vi "GestureOLED.vi"() -> ()   [LabVIEW 2024]
uses:
  Driver/Public/Digital Pull Direction.ctl
  4ccb7be8-d2ac-470e-b164-43973984285f.vi
  4331f14a-4e11-4a16-bb0d-2e9d18c5c6a1.vi
  51c12f6e-4a21-4d98-9fb3-1a2e6b8270e3.vi
  d8ff4ad1-6435-4902-b67c-6ac0edf8525d.vi
  64x128OLED/Public/InitialiseOLED.vi
  64x128OLED/Public/GetPicture.vi
  64x128OLED/Public/BuildMessagesFromPicture.vi
  Driver/CTIPicoVISA.lvlib
  64x128OLED/OLEDI2CMessageGenerator.lvlib
panel:
  out "Stopped":bool
  out "Numeric":i32
  out "2D Picture":picture
  out "loop":i32
  out "Identity":T1
  out "Init Data":string
  in  "stop":bool
  in  "VISA resource name in":refnum<visa-resource-name>="COM7"
  out "error out":errorcluster
  # "https://www.seeedstudio.com/Grove-Gesture-PAJ7620U2.html"
  # "https://wiki.seeedstudio.com/Grove-OLED-Display-0.96-SSD1315/"
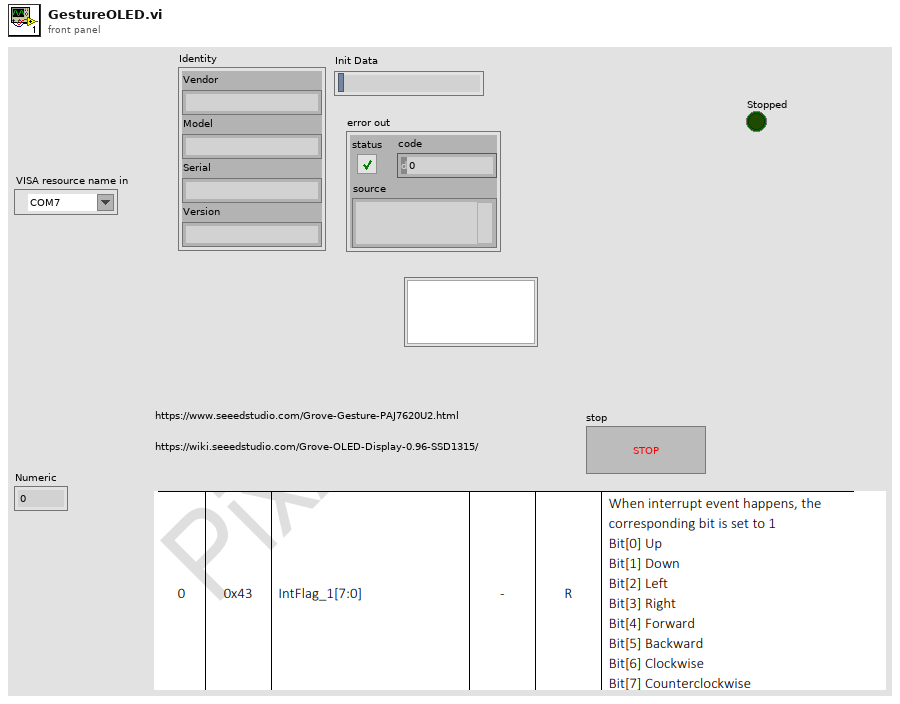
[diagram p1: front panel]
types:
  T1 = cluster{"Vendor":string, "Model":string, "Serial":string, "Version":string}
  T2 = cluster{"image type":i32, "image depth":i32, "image":u8[], "mask":u8[], "colors":u32[], "Rectangle":cluster{"left":i16, "top":i16, "right":i16, "bottom":i16}}
  T3 = typedef "CTIPicoVISA.lvlib/Digital Pull Direction.ctl" = enum16{"None", "Up", "Down", "Both"}
  T4 = cluster{"image type":i32, "image depth":i32, "image":u8[], "mask":u8[], "colors":u32[], "Rectangle":cluster{"left":i16, "top":i16, "right":i16, "bottom":i16}}[]
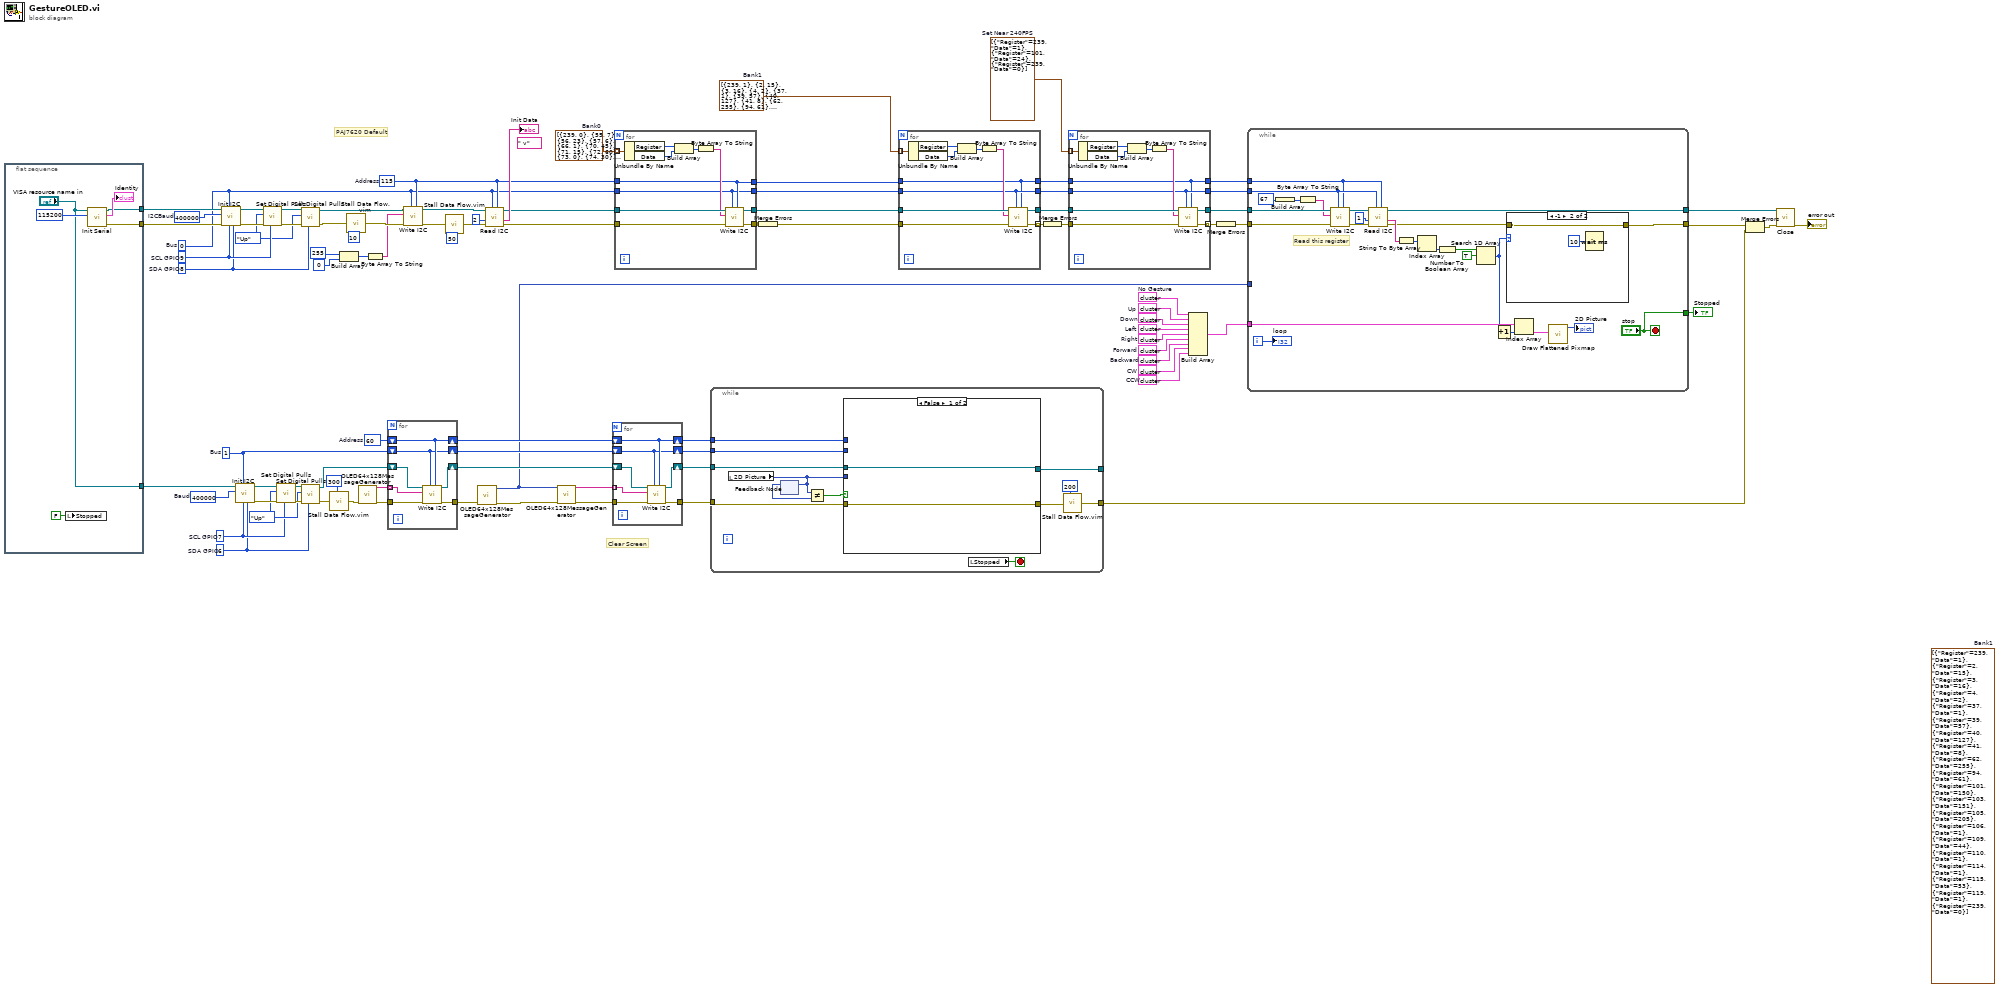
[diagram p0: block diagram]
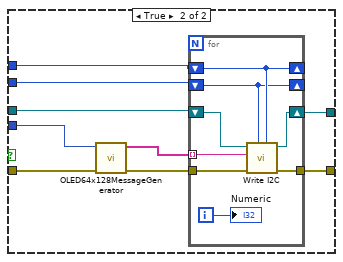
[diagram p2: hidden frame]
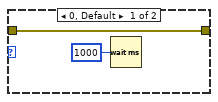
[diagram p3: hidden frame]
diagram:
  w1 = T2 {"image type"=0, "image depth"=8, "image"=array[8192 elements], "mask"=[], "colors"=[16777215, 15461356, 16579836, 11513775, 8158332, 13421772, 13816530, 0, 921102, 15329769, 8553090, 3421236, 15461355, 14935011, 1447446, 10000536, 1052688, 14803425, 15921906, 15000804, 13684944, 15856113, 16645629, 15658734, 3552822, 4079166, 11119017, 8289918, 4276545, 1052687, 395014, 7829367, 12171705, 15527148, 11645361, 65793, 131586, 2763306, 10987431, 16119285, 16316664, 6316128, 197379, 6447714, 14277081, 13158600, 6645093, 11316396, 13224393, 11184810, 6250335, 263172, 2171169, 13948116, 8092539, 10066329, 16250871, 12829635, 6118749, 2434341, 14013909, 16711422, 13750737, 8816262, 9868950, 14869218, 9474192, 4144959, 10658466, 3750201, 4934475, 15987699, 10724259, 328965, 9934743, 15790320, 12237498, 5592405, 15263976, 16185078, 6842472, 789516, 13487565, 7763574, 3815994, 16382457, 16514043, 5921370, 789515, 13092807, 12566463, 3684408, 12632256, 3355443, 11053224, 15592941, 14737632, 14145495, 5197647, 7697781, 14540253, 9408399, 16448250, 12698049, 12369084, 11579568, 14474460, 1644825, 5131854, 15066597, 3158320, 14671839, 4539717, 13355979, 13027014, 11382189, 10197915, 7105644, 15724527, 6974058, 7960953, 9276813, 8026746, 9342606, 4210752, 12303291, 11250603, 13882323, 11776947, 9013641, 8355711, 8882055, 11711154, 15527405, 14343133, 13553358, 14342874, 1907997, 7434609, 394758, 2368548, 5460819, 6710886, 4605510, 6776679, 12895428, 657930, 2302755, 5066061, 4473924, 3158064, 8618883, 2236962, 9079434, 4408131, 14079702, 13290186, 9211020, 7039851, 13619151, 5789784, 4342338, 5987163, 460551, 6513507, 855309, 5000268, 1315860, 12040119, 5526612, 9539985, 4802889, 12105912, 3092271, 986895, 8224125, 9605778, 2829099, 1776411, 7566195, 1381653, 2500134, 15395562, 0, 0, 0, 0, 0, 0, 0, 0, 0, 0, 0, 0, 0, 0, 0, 0, 0, 0, 0, 0, 0, 0, 0, 0, 0, 0, 0, 0, 0, 0, 0, 0, 0, 0, 0, 0, 0, 0, 0, 0, 0, 0, 0, 0, 0, 0, 0, 0, 0, 0, 0, 0, 0, 0, 0, 0, 0, 0, 0, 0, 0, 0, 0, 0, 0, 0, 0, 0, 0, 0, 0, 0, 0], "Rectangle"={"left"=0, "top"=0, "right"=128, "bottom"=64}}  # CCW
  w2 = T2 {"image type"=0, "image depth"=8, "image"=array[8192 elements], "mask"=[], "colors"=[16777215, 15461356, 13421772, 8158332, 11513775, 16579836, 15329769, 921102, 0, 13816530, 15461355, 3421236, 8553090, 10000536, 1447446, 14935011, 16645629, 15856113, 13684944, 15000804, 15921906, 14803425, 1052688, 15527148, 12171705, 7829367, 4079166, 395014, 1052687, 4276545, 8289918, 11119017, 3552822, 15658734, 16119285, 10987431, 2763306, 131586, 65793, 11645361, 14277081, 6447714, 197379, 6316128, 16316664, 13948116, 2171169, 263172, 6250335, 11184810, 13224393, 13158600, 11316396, 6645093, 14013909, 2434341, 6118749, 12829635, 16250871, 10066329, 8092539, 4144959, 9474192, 14869218, 9868950, 8816262, 13750737, 16711422, 9934743, 328965, 10724259, 15987699, 4934475, 3750201, 10658466, 789516, 6842472, 16185078, 15263976, 5592405, 12237498, 15790320, 16382457, 3815994, 7763574, 13487565, 5921370, 16514043, 13092807, 789515, 12566463, 12632256, 3684408, 3355443, 15592941, 11053224, 7697781, 5197647, 14145495, 14737632, 12698049, 16448250, 9408399, 14540253, 5131854, 1644825, 14474460, 11579568, 12369084, 13355979, 4539717, 14671839, 3158320, 15066597, 10197915, 11382189, 13027014, 6974058, 15724527, 7105644, 9342606, 8026746, 9276813, 7960953, 12303291, 4210752, 11250603, 11711154, 8882055, 8355711, 9013641, 11776947, 13882323, 15527405, 14343133, 1907997, 8750469, 14342874, 6776679, 12895428, 7368816, 3092271, 8947848, 3618615, 5066061, 12040119, 4802889, 5789784, 5723991, 526344, 14079702, 13290186, 3487029, 13619151, 9803157, 14408667, 394758, 460551, 4408131, 2894892, 5000268, 986895, 5658198, 12105912, 6513507, 7566195, 1973790, 5526612, 2829099, 1776411, 15395562, 0, 0, 0, 0, 0, 0, 0, 0, 0, 0, 0, 0, 0, 0, 0, 0, 0, 0, 0, 0, 0, 0, 0, 0, 0, 0, 0, 0, 0, 0, 0, 0, 0, 0, 0, 0, 0, 0, 0, 0, 0, 0, 0, 0, 0, 0, 0, 0, 0, 0, 0, 0, 0, 0, 0, 0, 0, 0, 0, 0, 0, 0, 0, 0, 0, 0, 0, 0, 0, 0, 0, 0, 0, 0, 0, 0, 0, 0, 0, 0, 0, 0, 0, 0, 0], "Rectangle"={"left"=0, "top"=0, "right"=128, "bottom"=64}}  # CW
  w3 = T2 {"image type"=0, "image depth"=8, "image"=array[8192 elements], "mask"=[], "colors"=[16777215, 16250871, 15724527, 14935011, 14079702, 13421772, 12961221, 15000804, 15921906, 14145495, 11842740, 9342606, 6381921, 3026478, 0, 2960685, 6447714, 9408399, 15395562, 8092539, 3421236, 3487029, 8026746, 11645361, 5066061, 256, 11579568, 16514043, 6513507, 13487565, 16514299, 15856113, 10658466, 1118481, 263172, 263428, 1052944, 10724259, 8684676, 131586, 15198183, 7434609, 65793, 7368816, 723979, 6513763, 2631976, 10066585, 12237754, 12171961, 12171960, 4539973, 14935267, 4605766, 9013640, 15790320, 9013641, 9211275, 15987699, 15987955, 9277068, 11776947, 9803156, 16119285, 16316664, 262916, 10527135, 16382457, 10790308, 11053480, 11776946, 16645885, 16711422, 11908789, 12040375, 2434597, 10198170, 12895683, 12895684, 13224649, 16711678, 13224393, 12961476, 10395550, 2566184, 4934731, 15066596, 13619407, 13422028, 16382456, 16316920, 13487564, 13684943, 15066597, 9013897, 13882579, 13553613, 13488077, 13816529, 9671571, 16185078, 9868950, 10724258, 16448250, 11316396, 16579835, 197379, 11908532, 11777203, 12369083, 12566463, 12763841, 132098, 7960953, 2698025, 13092806, 13092807, 3026733, 328965, 3224112, 10395806, 10527136, 3421492, 328709, 6513251, 986895, 16579836, 8618883, 7303023, 15329769, 15132390, 657930, 1118737, 3026477, 14211288, 13355979, 14013909, 16645629, 5658198, 1513239, 8224125, 5526612, 2434341, 7039851, 13027014, 4868682, 394758, 11447982, 9276813, 10066329, 16053492, 9539985, 7500402, 10526880, 4079166, 6974058, 11908533, 12303291, 6908265, 2894892, 3684408, 14869218, 2171169, 4737096, 3552822, 3355443, 3881787, 3815994, 15658734, 14606046, 5723991, 3750201, 2565927, 10329501, 10263708, 10855845, 7895160, 8882055, 13816530, 8487297, 13684944, 2829099, 1842204, 4013373, 6579300, 1447446, 8750469, 5131854, 2368548, 3618615, 10461087, 9474192, 14277081, 11184810, 1315860, 6184542, 8947848, 789516, 7763574, 1381653, 12763842, 12105912, 5987163, 1579032, 6776679, 15527148, 1907997, 0, 0, 0, 0, 0, 0, 0, 0, 0, 0, 0, 0, 0, 0, 0, 0, 0, 0, 0, 0, 0, 0, 0, 0, 0, 0, 0, 0, 0, 0, 0, 0, 0, 0, 0, 0, 0, 0, 0, 0, 0, 0, 0, 0, 0, 0, 0, 0, 0], "Rectangle"={"left"=0, "top"=0, "right"=128, "bottom"=64}}  # Backward
  w4 = T2 {"image type"=0, "image depth"=8, "image"=array[8192 elements], "mask"=[], "colors"=[16777215, 16250871, 15724527, 15000804, 14079702, 13421772, 12961221, 13355979, 14013909, 14935011, 15921906, 14145495, 11842740, 9408399, 6447714, 3026477, 0, 3026478, 9342606, 14211288, 15395562, 8026746, 3487029, 3421236, 11645361, 5066061, 16514043, 13487565, 6513507, 15856113, 10724259, 657930, 263172, 1118737, 10658466, 8684676, 131586, 8618883, 15329769, 15198183, 7368816, 65793, 7303023, 15132390, 16579836, 256, 1118481, 986895, 6513251, 11579568, 197379, 328965, 3224112, 10395806, 10527136, 3421492, 328709, 2698025, 13092806, 13092807, 3026733, 12566463, 12763841, 132098, 7960953, 12369083, 16711422, 11908532, 11777203, 11776947, 11316396, 16579835, 10724258, 16448250, 6381921, 2960685, 10066585, 9868950, 9671571, 16185078, 9013897, 13882579, 13553613, 13488077, 13816529, 9013641, 4934731, 15066596, 13619407, 13422028, 16382456, 16316920, 13487564, 13684943, 15066597, 2434597, 10198170, 12895683, 12895684, 11908789, 13224649, 16711678, 13224393, 12961476, 10395550, 2566184, 12040375, 11776946, 16645885, 11053480, 16514299, 10527135, 16382457, 10790308, 9803156, 16119285, 16316664, 262916, 9211275, 15987699, 15987955, 9277068, 9013640, 15790320, 4539973, 14935267, 4605766, 2631976, 12237754, 12171961, 12171960, 6513763, 723979, 7434609, 263428, 1052944, 8092539, 16645629, 15263976, 1776411, 5658198, 6052956, 3355443, 2434341, 15527148, 5395026, 10197915, 7105644, 9474192, 15461355, 8750469, 8553090, 8289918, 8882055, 11908533, 7895160, 3618615, 12698049, 7039851, 4013373, 11053224, 723723, 5329233, 1315860, 1513239, 14671839, 12829635, 3289650, 5460819, 14606046, 11513775, 2763306, 7566195, 6776679, 5921370, 3552822, 5855577, 5789784, 921102, 7171437, 7237230, 11184810, 2368548, 7763574, 13027014, 4276545, 15658734, 1579032, 14803425, 1907997, 2565927, 6579300, 10855845, 11711154, 6908265, 3750201, 8224125, 8816262, 2500134, 10921638, 460551, 6316128, 6118749, 5723991, 14277081, 12632256, 7829367, 2631720, 1644825, 10329501, 4934475, 14474460, 3947580, 4539717, 10132122, 1710618, 5592405, 14737632, 5131854, 10790052, 526344, 4605510, 3815994, 12303291, 2894892, 3881787, 4079166, 5197647, 6184542, 10987431, 12040119, 9737364, 855309, 10000536, 4737096, 13750737, 789516, 5000268, 8355711, 0, 0, 0, 0, 0, 0, 0, 0, 0, 0, 0, 0, 0, 0, 0, 0, 0], "Rectangle"={"left"=0, "top"=0, "right"=128, "bottom"=64}}  # Forward
  w6 = T2 {"image type"=0, "image depth"=24, "image"=array[24576 elements], "mask"=[], "colors"=[], "Rectangle"={"left"=0, "top"=0, "right"=128, "bottom"=64}}  # Right
  w7 = T2 {"image type"=0, "image depth"=24, "image"=array[24576 elements], "mask"=[], "colors"=[], "Rectangle"={"left"=0, "top"=0, "right"=128, "bottom"=64}}  # Left
  w8 = T2 {"image type"=0, "image depth"=24, "image"=array[24576 elements], "mask"=[], "colors"=[], "Rectangle"={"left"=0, "top"=0, "right"=128, "bottom"=64}}  # Down
  w9 = T2 {"image type"=0, "image depth"=24, "image"=array[24576 elements], "mask"=[], "colors"=[], "Rectangle"={"left"=0, "top"=0, "right"=128, "bottom"=64}}  # Up
  w10 = T2 {"image type"=0, "image depth"=8, "image"=array[8192 elements], "mask"=[], "colors"=[16777215, 16645629, 14869218, 7237230, 16579836, 14342874, 15592941, 11316396, 3750201, 10395294, 1776411, 5921370, 11250603, 16514043, 7500402, 6513507, 11447982, 13619151, 11776947, 0, 13158600, 5592405, 13224393, 15790320, 12171705, 16711422, 5658198, 14474460, 15658734, 5789784, 2368548, 13948116, 14277081, 13882323, 8750469, 8421504, 16316664, 12237498, 12369084, 14935011, 12105912, 11711154, 12763842, 15066597, 12303291, 11579568, 13421772, 9737364, 9803157, 15198183, 4671303, 13750737, 12434877, 16382457, 5329233, 4737096, 5460819, 5723991, 15856113, 16448250, 11053224, 14540253, 12698049, 13027014, 6250335, 13487565, 131586, 7105644, 65793, 1907997, 13355979, 15921906, 8816262, 11184810, 460551, 4473924, 5131854, 4013373, 14079702, 723723, 8553090, 11513775, 11842740, 5395026, 13816530, 10790052, 8487297, 4539717, 1315860, 2302755, 6184542, 16119285, 9539985, 2434341, 5263440, 13290186, 15000804, 9211020, 6447714, 7434609, 12566463, 6842472, 9934743, 11645361, 6579300, 6381921, 3618615, 10658466, 15461355, 6710886, 6974058, 7895160, 11119017, 11974326, 10855845, 13092807, 263172, 8947848, 9145227, 4802889, 1842204, 15527148, 6645093, 15132390, 4868682, 10724259, 9474192, 15987699, 7631988, 2500134, 16250871, 197379, 5987163, 4079166, 3552822, 13553358, 4408131, 1513239, 328965, 5066061, 7697781, 4934475, 394758, 789516, 1052688, 1381653, 9868950, 12500670, 2171169, 2236962, 1579032, 1973790, 15263976, 10197915, 1447446, 2565927, 3026478, 8882055, 7303023, 14013909, 6908265, 14211288, 5000268, 12632256, 14803425, 14606046, 15395562, 7171437, 1250067, 15724527, 4605510, 4342338, 7566195, 9013641, 10263708, 15329769, 8092539, 14737632, 8684676, 13684944, 7368816, 11908533, 11382189, 4276545, 5197647, 6052956, 9079434, 4210752, 2631720, 526344, 8026746, 3684408, 3487029, 9408399, 3947580, 12961221, 4144959, 2894892, 7039851, 8618883, 3289650, 8289918, 10987431, 5526612, 3815994, 3223857, 2697513, 9342606, 16053492, 3881787, 1644825, 10132122, 3355443, 10066329, 2105376, 1710618, 10461087, 5855577, 1184274, 12829635, 921102, 2039583, 2829099, 657930, 1118481, 2763306, 8158332, 855309, 10921638, 14671839, 0, 0, 0, 0, 0, 0, 0, 0, 0, 0, 0, 0, 0, 0, 0, 0, 0, 0, 0, 0, 0, 0, 0, 0, 0, 0], "Rectangle"={"left"=0, "top"=0, "right"=128, "bottom"=64}}  # No Gesture
  w46 = u8 0  # Bus
  w72 = 8  # SDA GPIO
  w74 = 9  # SCL GPIO
  w35 = u8 1  # Bus
  w31 = 6  # SDA GPIO
  w32 = 7  # SCL GPIO
  w40 = Digital_Pull_Direction."Up" ("Pull")
  w34 = u8 60  # Address
  w37 = u32 400000  # Baud
  (unwired) cluster{"Register":u8, "Data":u8}[] [{"Register"=239, "Data"=1}, {"Register"=2, "Data"=15}, {"Register"=3, "Data"=16}, {"Register"=4, "Data"=2}, {"Register"=37, "Data"=1}, {"Register"=39, "Data"=57}, {"Register"=40, "Data"=127}, {"Register"=41, "Data"=8}, {"Register"=62, "Data"=255}, {"Register"=94, "Data"=61}, {"Register"=101, "Data"=150}, {"Register"=103, "Data"=151}, {"Register"=105, "Data"=205}, {"Register"=106, "Data"=1}, {"Register"=109, "Data"=44}, {"Register"=110, "Data"=1}, {"Register"=114, "Data"=1}, {"Register"=115, "Data"=53}, {"Register"=119, "Data"=1}, {"Register"=239, "Data"=0}]  # Bank1
  w53 = cluster{"Register":u8, "Data":u8}[] [{"Register"=239, "Data"=1}, {"Register"=101, "Data"=24}, {"Register"=239, "Data"=0}]  # Set Near 240FPS
  w62 = cluster{"Register":u8, "Data":u8}[] [{"Register"=239, "Data"=1}, {"Register"=2, "Data"=15}, {"Register"=3, "Data"=16}, {"Register"=4, "Data"=2}, {"Register"=37, "Data"=1}, {"Register"=39, "Data"=57}, {"Register"=40, "Data"=127}, {"Register"=41, "Data"=8}, {"Register"=62, "Data"=255}, {"Register"=94, "Data"=61}, {"Register"=101, "Data"=150}, {"Register"=103, "Data"=151}, {"Register"=105, "Data"=205}, {"Register"=106, "Data"=1}, {"Register"=109, "Data"=44}, {"Register"=110, "Data"=1}, {"Register"=114, "Data"=1}, {"Register"=115, "Data"=53}, {"Register"=119, "Data"=1}, {"Register"=239, "Data"=0}]  # Bank1
  w69 = cluster{"Register":u8, "Data":u8}[] [{"Register"=239, "Data"=0}, {"Register"=55, "Data"=7}, {"Register"=56, "Data"=23}, {"Register"=57, "Data"=6}, {"Register"=66, "Data"=1}, {"Register"=70, "Data"=45}, {"Register"=71, "Data"=15}, {"Register"=72, "Data"=60}, {"Register"=73, "Data"=0}, {"Register"=74, "Data"=30}, {"Register"=76, "Data"=32}, {"Register"=81, "Data"=16}, {"Register"=94, "Data"=16}, {"Register"=96, "Data"=39}, {"Register"=128, "Data"=66}, {"Register"=129, "Data"=68}, {"Register"=130, "Data"=4}, {"Register"=139, "Data"=1}, {"Register"=144, "Data"=6}, {"Register"=149, "Data"=10}, {"Register"=150, "Data"=12}, {"Register"=151, "Data"=5}, {"Register"=154, "Data"=20}, {"Register"=156, "Data"=63}, {"Register"=165, "Data"=25}, {"Register"=204, "Data"=25}, {"Register"=205, "Data"=11}, {"Register"=206, "Data"=19}, {"Register"=207, "Data"=100}, {"Register"=208, "Data"=33}]  # Bank0
  (unwired) " v" ("Init Data")
  w73 = Digital_Pull_Direction."Up" ("Pull")
  w66 = u8 115  # Address
  w91 = u32 400000  # I2CBaud
  # "Clear Screen"
  # "PAJ7620 Default"
  n1 = flat-sequence {
    tunnel: [w95] -> w58
    tunnel: [w94] -> w57
    tunnel: ["VISA resource name in"] -> w18
    frame #0 {
      n2 = local write "Stopped"(FALSE ("Stopped")) -> ()
      n3 = call "Init Serial.vi"("Baud (115200)"=u32 115200, "VISA resource name in"="VISA resource name in") -> ("error out"=w94:errorcluster, "Identity"=→"Identity":T1, "VISA resource name Out"=w95:refnum<visa-resource-name>)  [unwired: 7 in]
    }
  }
  n4 = call "Init I2C.vi"("SDA GPIO"=w72, "SCL GPIO"=w74, "Bus"=w46, "error in (no error)"=w57, "Baud"=w91, "VISA resource name in"=w58) -> ("error out"=w77:errorcluster, "VISA resource name"=w78:refnum<visa-resource-name>)  [unwired: 4 in]
  n5 = call "Init I2C.vi"("SDA GPIO"=w31, "SCL GPIO"=w32, "Bus"=w35, "Baud"=w37, "VISA resource name in"=w18) -> ("error out"=w43:errorcluster, "VISA resource name"=w44:refnum<visa-resource-name>)  [unwired: 5 in]
  n6 = call "Set Digital Pulls.vi"("GPIO"=w74, "error in (no error)"=w77, "Pull"=w73, "VISA resource name in"=w78) -> ("error out"=w75:errorcluster, "VISA resource name"=w76:refnum<visa-resource-name>)  [unwired: 6 in]
  n7 = call "Set Digital Pulls.vi"("GPIO"=w32, "error in (no error)"=w43, "Pull"=w40, "VISA resource name in"=w44) -> ("error out"=w41:errorcluster, "VISA resource name"=w42:refnum<visa-resource-name>)  [unwired: 6 in]
  n8 = call "Set Digital Pulls.vi"("GPIO"=w72, "error in (no error)"=w75, "Pull"=w73, "VISA resource name in"=w76) -> ("error out"=w70:errorcluster, "VISA resource name"=w71:refnum<visa-resource-name>)  [unwired: 6 in]
  n9 = call "Set Digital Pulls.vi"("GPIO"=w31, "error in (no error)"=w41, "Pull"=w40, "VISA resource name in"=w42) -> ("error out"=w29:errorcluster, "VISA resource name"=w28:refnum<visa-resource-name>)  [unwired: 6 in]
  n10 = call "Stall Data Flow.vim"("value in"=w29, "milliseconds to wait"=u32 300) -> ("value out"=w38:errorcluster)  [unwired: 1 out]
  n11 = Build Array(u8 255 ("Value"), u8 0 ("Value")) -> (w89:u8[])
  n12 = call "Stall Data Flow.vim"("value in"=w70, "milliseconds to wait"=u32 10) -> ("value out"=w86:errorcluster)  [unwired: 1 out]
  n13 = call-poly "OLED64x128MessageGenerator.vi"("error in (no error)"=w38) -> ("error out"=w36:errorcluster, "Messages"=w45:string[])  [unwired: 9 in]
  n14 = Byte Array To String(unsigned byte array=w89) -> (string=w85:string)
  n15 = for {
    tunnel: w45 -> [w102] mode=indexing
    tunnel: w36 -> [w104]
    tunnel: [w101] -> w33
    shift-right: [w100] -> w23
    shift-left: w28 -> [w103]
    shift-right: [w99] -> w24
    shift-left: w34 -> [w99]
    shift-right: [w98] -> w22
    shift-left: w35 -> [w98]
    n16 = call "Write I2C.vi"("Address"=w99, "Bus"=w98, "error in (no error)"=w104, "Data"=w102, "VISA resource name in"=w103) -> ("error out"=w101:errorcluster, "VISA resource name"=w100:refnum<visa-resource-name>)  [unwired: 5 in]
  }
  n17 = call "Write I2C.vi"("Address"=w66, "Bus"=w46, "error in (no error)"=w86, "Data"=w85, "VISA resource name in"=w71) -> ("error out"=w83:errorcluster, "VISA resource name"=w82:refnum<visa-resource-name>)  [unwired: 5 in]
  n18 = call "Stall Data Flow.vim"("value in"=w83, "milliseconds to wait"=u32 50) -> ("value out"=w81:errorcluster)  [unwired: 1 out]
  n19 = call-poly "OLED64x128MessageGenerator.vi"("error in (no error)"=w33) -> ("error out"=w30:errorcluster, "2D Picture"=w17:picture)  [unwired: 9 in]
  n20 = call "Read I2C.vi"("Address"=w66, "Bus"=w46, "error in (no error)"=w81, "Len"=u8 2, "VISA resource name in"=w82) -> ("error out"=w68:errorcluster, "Data"=→"Init Data":string, "VISA resource name"=w67:refnum<visa-resource-name>)  [unwired: 4 in]
  n21 = call-poly "OLED64x128MessageGenerator.vi"("error in (no error)"=w30, "2D Picture"=w17) -> ("error out"=w27:errorcluster, "Messages"=w26:string[])  [unwired: 8 in]
  n22 = for {
    tunnel: w26 -> [w109] mode=indexing
    tunnel: w27 -> [w111]
    tunnel: [w108] -> w25
    shift-right: [w107] -> w21
    shift-left: w23 -> [w110]
    shift-right: [w106] -> w19
    shift-left: w24 -> [w106]
    shift-right: [w105] -> w20
    shift-left: w22 -> [w105]
    n23 = call "Write I2C.vi"("Address"=w106, "Bus"=w105, "error in (no error)"=w111, "Data"=w109, "VISA resource name in"=w110) -> ("error out"=w108:errorcluster, "VISA resource name"=w107:refnum<visa-resource-name>)  [unwired: 5 in]
  }
  n24 = for {
    tunnel: w69 -> [w119] mode=indexing
    tunnel: w68 -> [w121]
    tunnel: w67 -> [w122]
    tunnel: w46 -> [w112]
    tunnel: w66 -> [w113]
    tunnel: [w115] -> w65
    tunnel: [w114] -> _ mode=indexing
    tunnel: [w114] -> w64
    tunnel: [w113] -> w60
    tunnel: [w112] -> w59
    n25 = Unbundle By Name(w119) -> ("Register"=w118:u8, "Data"=w117:u8)
    n26 = Build Array(w118, w117) -> (w120:u8[])
    n27 = Byte Array To String(unsigned byte array=w120) -> (string=w116:string)
    n28 = call "Write I2C.vi"("Address"=w113, "Bus"=w112, "error in (no error)"=w121, "Data"=w116, "VISA resource name in"=w122) -> ("error out"=w114:errorcluster, "VISA resource name"=w115:refnum<visa-resource-name>)  [unwired: 5 in]
  }
  n29 = while {
    tunnel: w25 -> [w134]
    tunnel: w19 -> [w133]
    tunnel: w20 -> [w132]
    tunnel: w21 -> [w131]
    tunnel: [w130] -> _
    tunnel: [w127] -> w12
    stop <- w126 stop-if-true
    n30 = local read "2D Picture"() -> (w123:picture)
    n31 = feedback-in #1(w123) -> ()
    n32 = feedback #1() -> (w125:picture)  [unwired: 1 in]
    n33 = Not Equal?(x=w123, y=w125) -> (x != y?=w124:bool)
    n34 = case shown="False" w124 {
      tunnel: w134 -> [w135 w145]
      tunnel: w133 -> [_ w144]
      tunnel: w132 -> [_ w143]
      tunnel: w131 -> [w136 w142]
      tunnel: [w136 w139] -> w130
      tunnel: [w135 w138] -> w128
      tunnel: w123 -> [_ w137]
      frame False {
      }
      frame True {
        n35 = call-poly "OLED64x128MessageGenerator.vi"("error in (no error)"=w145, "2D Picture"=w137) -> ("error out"=w141:errorcluster, "Messages"=w140:string[])  [unwired: 8 in]
        n36 = for {
          tunnel: w140 -> [w151] mode=indexing
          tunnel: w141 -> [w153]
          tunnel: [w150] -> w138
          shift-right: [w149] -> w139
          shift-left: w142 -> [w152]
          shift-right: [w148] -> _
          shift-left: w144 -> [w148]
          shift-right: [w147] -> _
          shift-left: w143 -> [w147]
          i -> [w146]
          n37 = call "Write I2C.vi"("Address"=w148, "Bus"=w147, "error in (no error)"=w153, "Data"=w151, "VISA resource name in"=w152) -> ("error out"=w150:errorcluster, "VISA resource name"=w149:refnum<visa-resource-name>)  [unwired: 5 in]
          "Numeric" <- w146
        }
      }
    }
    n38 = local read "Stopped"() -> (w126:bool)
    n39 = call "Stall Data Flow.vim"("value in"=w128, "milliseconds to wait"=u32 200) -> ("value out"=w127:errorcluster)  [unwired: 1 out]
  }
  n40 = Merge Errors(w64) -> (w63:errorcluster)
  n41 = for {
    tunnel: w62 -> [w161] mode=indexing
    tunnel: w63 -> [w163]
    tunnel: w65 -> [w164]
    tunnel: w59 -> [w155]
    tunnel: w60 -> [w154]
    tunnel: [w157] -> w55
    tunnel: [w156] -> w61 mode=indexing
    tunnel: [w155] -> w54
    tunnel: [w154] -> w52
    n42 = Unbundle By Name(w161) -> ("Register"=w160:u8, "Data"=w159:u8)
    n43 = Build Array(w160, w159) -> (w162:u8[])
    n44 = Byte Array To String(unsigned byte array=w162) -> (string=w158:string)
    n45 = call "Write I2C.vi"("Address"=w154, "Bus"=w155, "error in (no error)"=w163, "Data"=w158, "VISA resource name in"=w164) -> ("error out"=w156:errorcluster, "VISA resource name"=w157:refnum<visa-resource-name>)  [unwired: 5 in]
  }
  n46 = Merge Errors(w61) -> (w56:errorcluster)
  n47 = for {
    tunnel: w53 -> [w172] mode=indexing
    tunnel: w56 -> [w174]
    tunnel: w55 -> [w175]
    tunnel: w54 -> [w166]
    tunnel: w52 -> [w165]
    tunnel: [w168] -> w49
    tunnel: [w167] -> w51 mode=indexing
    tunnel: [w166] -> w48
    tunnel: [w165] -> w47
    n48 = Unbundle By Name(w172) -> ("Register"=w171:u8, "Data"=w170:u8)
    n49 = Build Array(w171, w170) -> (w173:u8[])
    n50 = Byte Array To String(unsigned byte array=w173) -> (string=w169:string)
    n51 = call "Write I2C.vi"("Address"=w165, "Bus"=w166, "error in (no error)"=w174, "Data"=w169, "VISA resource name in"=w175) -> ("error out"=w167:errorcluster, "VISA resource name"=w168:refnum<visa-resource-name>)  [unwired: 5 in]
  }
  n52 = Build Array(w10, w9, w8, w7, w6, w4, w3, w2, w1) -> (w5:T4)
  n53 = Merge Errors(w51) -> (w50:errorcluster)
  n54 = while {
    tunnel: w50 -> [w195]
    tunnel: [w182] -> w16
    tunnel: w49 -> [w196]
    tunnel: [w200] -> w15
    tunnel: w48 -> [w192]
    tunnel: w47 -> [w191]
    tunnel: w17 -> [_]
    tunnel: ["stop"] -> w11
    tunnel: w5 -> [w180]
    i -> [w187]
    stop <- "stop" stop-if-true
    # "Read this register"
    n55 = Build Array(u8 67 ("Register")) -> (w190:u8[])
    n56 = Byte Array To String(unsigned byte array=w190) -> (string=w188:string)
    n57 = call "Write I2C.vi"("Address"=w191, "Bus"=w192, "error in (no error)"=w195, "Data"=w188, "VISA resource name in"=w196) -> ("error out"=w194:errorcluster, "VISA resource name"=w193:refnum<visa-resource-name>)  [unwired: 5 in]
    n58 = call "Read I2C.vi"("Address"=w191, "Bus"=w192, "error in (no error)"=w194, "Len"=u8 1, "VISA resource name in"=w193) -> ("error out"=w183:errorcluster, "Data"=w199:string, "VISA resource name"=w200:refnum<visa-resource-name>)  [unwired: 4 in]
    n59 = String To Byte Array(string=w199) -> (unsigned byte array=w198:u8[])
    n60 = Index Array(array=w198) -> (element=w197:u8)  [unwired: 1 in]
    n61 = Number To Boolean Array(number=w197) -> (Boolean array=w185:bool[])
    n62 = Search 1D Array(1D array=w185, element=TRUE) -> (index of element=w177:i32)  [unwired: 1 in]
    n63 = Increment(x=w177) -> (x+1=w176:i32)
    n64 = case shown="-1" w177 {
      tunnel: w183 -> [w201 w204]
      tunnel: [w201 w204] -> w182
      frame 0, Default {
        n65 = Wait (ms)(milliseconds to wait=u32 1000) -> ()  [unwired: 1 out]
      }
      frame -1 {
        n66 = Wait (ms)(milliseconds to wait=u32 10) -> ()  [unwired: 1 out]
      }
    }
    n67 = Index Array(array=w180, index=w176) -> (element=w179:T2)
    n68 = call <vilib>:"Draw Flattened Pixmap.vi"("image data"=w179) -> ("new picture"=→"2D Picture":picture)  [unwired: 8 in]
    "loop" <- w187
  }
  "Stopped" <- w11
  n69 = Merge Errors(w16, w12) -> (w13:errorcluster)
  n70 = call "Close.vi"("error in (no error)"=w13, "VISA resource name in"=w15) -> ("error out"=→"error out":errorcluster)  [unwired: 9 in]
